vi "Create Server.vi"(8 "error in (no error)":errorcluster, 9 "id":i32, 10 "New Server":T1, 11 "Variant in":variant) -> (0 "error out":errorcluster, 1 "Data Value Reference out":refnum<data-value>, 2 "unique server id out":i32, 3 "Variant":variant)   [LabVIEW 2025, in "MCP Server.lvlib"]
doc: "Initializes a new server and adds it to the variant lookup table."
uses:
  MCP Server.lvlib
  Server Data.ctl
  Tool Data.ctl
  Input Parameter.ctl
  Output Parameter.ctl
  Logging.ctl
  User Events.ctl
  onRpc.ctl
  Prompt Data.ctl
  Prompt Argument.ctl
  resource data.ctl
  <vilib>/IlluminatedG/IG HTTP Server/HTTP Server/Server/Server.lvclass
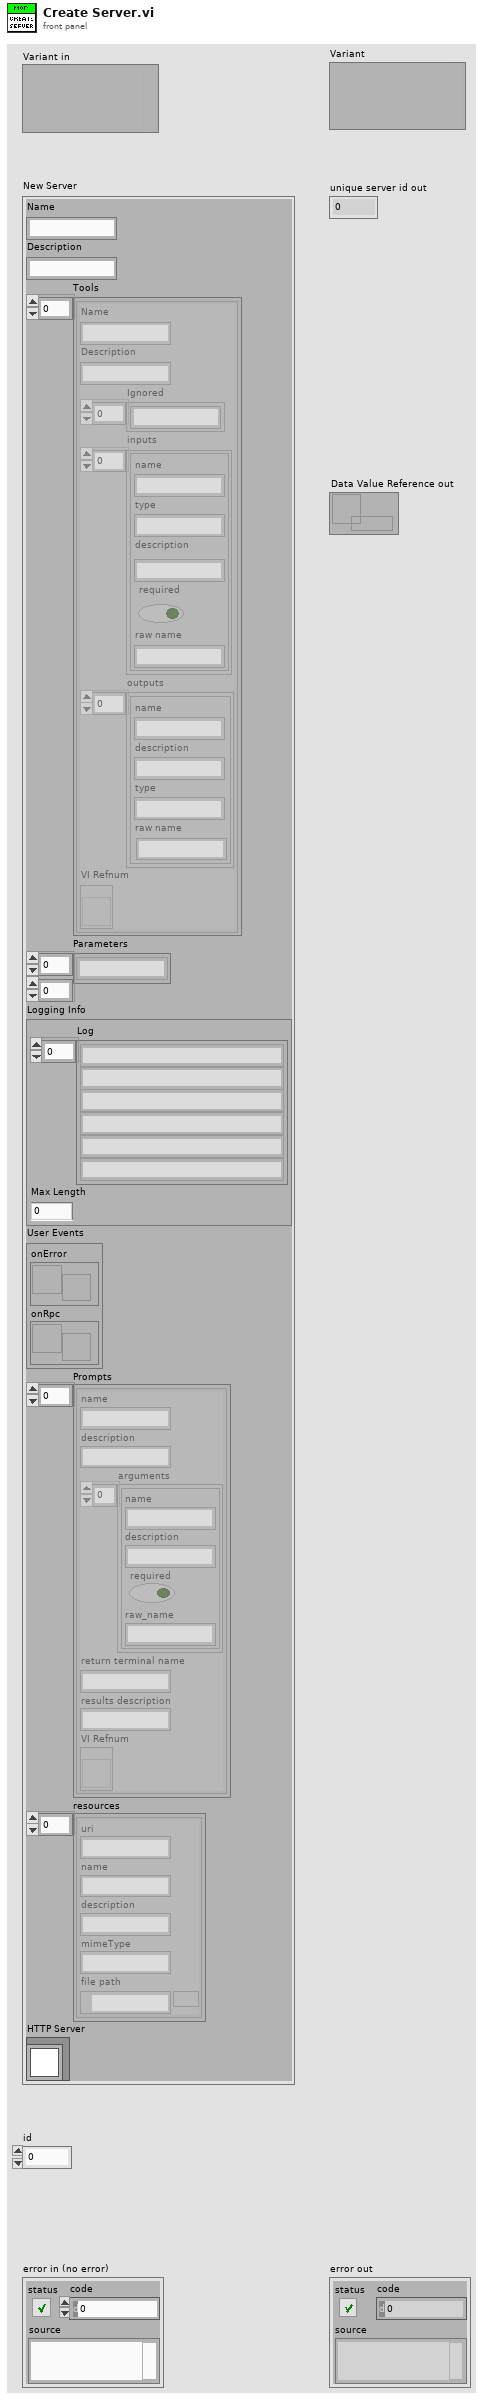
[diagram p1: front panel]
types:
  T1 = typedef "MCP Server.lvlib/Server Data.ctl" = cluster{"Name":string, "Description":string, "Tools":T2[], "Parameters":string[][], "Logging Info":T5, "User Events":T6, "Prompts":T7[], "resources":T9[], "HTTP Server":refnum<class "Server.lvclass">}
  T2 = typedef "MCP Server.lvlib/Tool Data.ctl" = cluster{"Name":string, "Description":string, "Ignored":string[], "inputs":T3[], "outputs":T4[], "VI Refnum":refnum<vi>}
  T3 = typedef "MCP Server.lvlib/Input Parameter.ctl" = cluster{"name":string, "type":string, "description":string, "required":bool, "raw name":string}
  T4 = typedef "MCP Server.lvlib/Output Parameter.ctl" = cluster{"name":string, "description":string, "type":string, "raw name":string}
  T5 = typedef "MCP Server.lvlib/Logging.ctl" = cluster{"Log":string[], "Max Length":i32}
  T6 = typedef "MCP Server.lvlib/User Events.ctl" = cluster{"onError":refnum<user-event>, "onRpc":refnum<user-event>}
  T7 = typedef "MCP Server.lvlib/Prompt Data.ctl" = cluster{"name":string, "description":string, "arguments":T8[], "return terminal name":string, "results description":string, "VI Refnum":refnum<vi>}
  T8 = typedef "MCP Server.lvlib/Prompt Argument.ctl" = cluster{"name":string, "description":string, "required":bool, "raw_name":string}
  T9 = typedef "MCP Server.lvlib/resource data.ctl" = cluster{"uri":string, "name":string, "description":string, "mimeType":string, "file path":path}
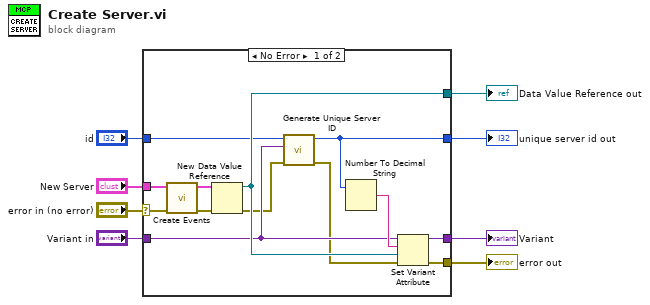
[diagram p0: block diagram]
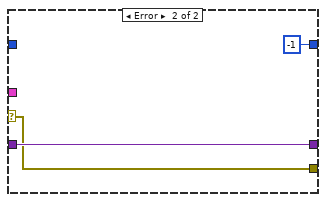
[diagram p2: hidden frame]
diagram:
  n1 = case shown="No Error" "error in (no error)" {
    selector: "error in (no error)" -> [w9 w23]
    tunnel: [w21 _] -> w8
    tunnel: [w19 -1 ("unique server id out")] -> w7
    tunnel: "Variant in" -> [w18 w24]
    tunnel: "id" -> [w17 _]
    tunnel: [w16 w23] -> w4
    tunnel: [w12 w24] -> w3
    tunnel: "New Server" -> [w11 _]
    frame No Error {
      n2 = call "Create Events.vi"("error in (no error)"=w9, "New Server in"=w11) -> ("error out"=w14:errorcluster, "New Server out"=w13:T1)  [unwired: 8 in]
      n3 = New Data Value Reference(data value=w13, error in=w14) -> (data value reference=w21:refnum<data-value>, error out=w15:errorcluster)
      n4 = call "Generate Unique Server ID.vi"("error in (no error)"=w15, "Variant"=w18, "server id in"=w17) -> ("error out"=w10:errorcluster, "unique server id out"=w19:i32)  [unwired: 7 in]
      n5 = Number To Decimal String(number=w19) -> (decimal integer string=w20:string)  [unwired: 1 in]
      n6 = Set Variant Attribute(Variant=w18, name=w20, value=w21, error in=w10) -> (Variant out=w12:variant, error out=w16:errorcluster)  [unwired: 1 out]
    }
    frame Error {
    }
  }
  "Data Value Reference out" <- w8
  "unique server id out" <- w7
  "error out" <- w4
  "Variant" <- w3
